vi "CRC计算.vi"(3 "需要检验的字符串（以16进制显示的字符串）":string) -> (0 "CRC校验位":string, 1 "字符长度":i32)   [LabVIEW 2015]
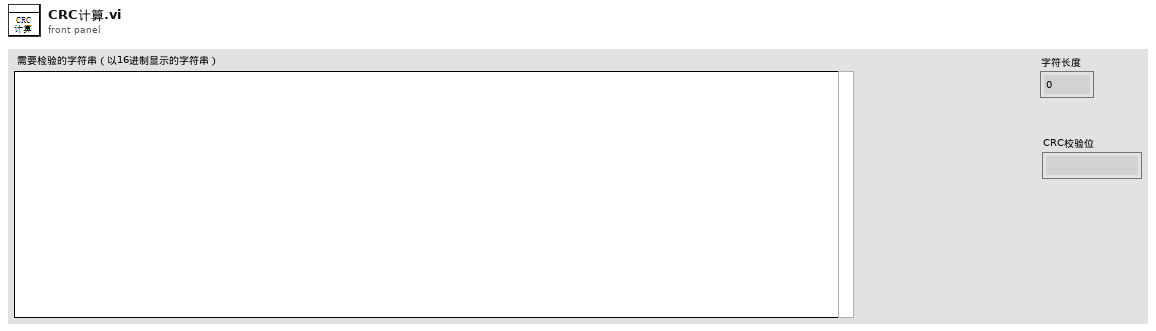
[diagram p1: front panel]
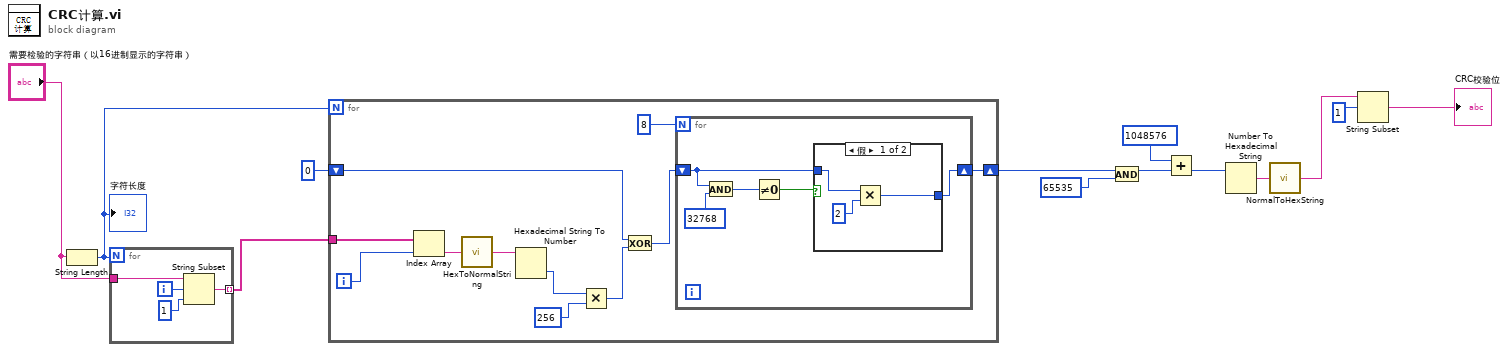
[diagram p0: block diagram]
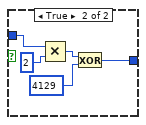
[diagram p2: hidden frame]
diagram:
  n1 = String Length(string="需要检验的字符串（以16进制显示的字符串）") -> (length=w10:i32)
  "字符长度" <- w10
  n2 = for {
    N: w10 -> [_]
    tunnel: "需要检验的字符串（以16进制显示的字符串）" -> [w17]
    tunnel: [w14] -> w12 mode=indexing
    i -> [w15]
    n3 = String Subset(string=w17, offset (0)=w15, length (rest)=1) -> (substring=w14:string)
  }
  n4 = for {
    N: w10 -> [_]
    tunnel: w12 -> [w28]
    shift-right: [w18] -> w9
    shift-left: 0 -> [w22]
    i -> [w27]
    n5 = Index Array(array=w28, index=w27) -> (element=w26:string)
    n6 = call "HexToNormalString.vi"("Hex Display"=w26) -> ("Normal Display"=w25:string)  [unwired: 14 in]
    n7 = Hexadecimal String To Number(string=w25) -> (number=w24:u32)  [unwired: 2 in, 1 out]
    n8 = Multiply(x=w24, y=256) -> (x*y=w21:u32)
    n9 = Exclusive Or(1:w21, 2:w22) -> (0:w19:u32)
    n10 = for {
      N: 8 -> [_]
      shift-right: [w29] -> w18
      shift-left: w19 -> [w30]
      n11 = And(x=w30, y=32768) -> (x .and. y?=w32:u32)
      n12 = Not Equal To 0?(x=w32) -> (x != 0?=w31:bool)
      n13 = case shown="假" w31 {
        tunnel: w30 -> [w36 w41]
        tunnel: [w34 w37] -> w29
        frame False {
          n14 = Multiply(x=w36, y=2) -> (x*y=w34:u32)
        }
        frame True {
          n15 = Multiply(x=w41, y=2) -> (x*y=w39:u32)
          n16 = Exclusive Or(1:4129, 2:w39) -> (0:w37:u32)
        }
      }
    }
  }
  n17 = And(x=w9, y=65535) -> (x .and. y?=w8:u32)
  n18 = Add(x=1048576, y=w8) -> (x+y=w5:u32)
  n19 = Number To Hexadecimal String(2:w5) -> (0:w6:string)  [unwired: 1 in]
  n20 = call "NormalToHexString.vi"("Normal Display String"=w6) -> ("Hex Display String"=w3:string)  [unwired: 14 in]
  n21 = String Subset(string=w3, offset (0)=1) -> (substring=→"CRC校验位":string)  [unwired: 1 in]
